vi "initializeKickForceValues.vi"(6 "samples":dbl, 7 "kickforce_min":dbl=1.0, 8 "error in (no error)":errorcluster, 9 "kickforce_max":dbl, 10 "delta":dbl, 11 "Game in":refnum<class "Game.lvclass">) -> (0 "error out":errorcluster, 2 "kickForceList":dbl[][](array[numeric]), 3 "Game out":refnum<class "Game.lvclass">)   [LabVIEW 2021, in "Game.lvclass"]
uses:
  Game.lvclass
  <vilib>/Analysis/1siggen.llb/Ramp Pattern by Delta.vi
  <vilib>/Analysis/NI_AALBase.lvlib
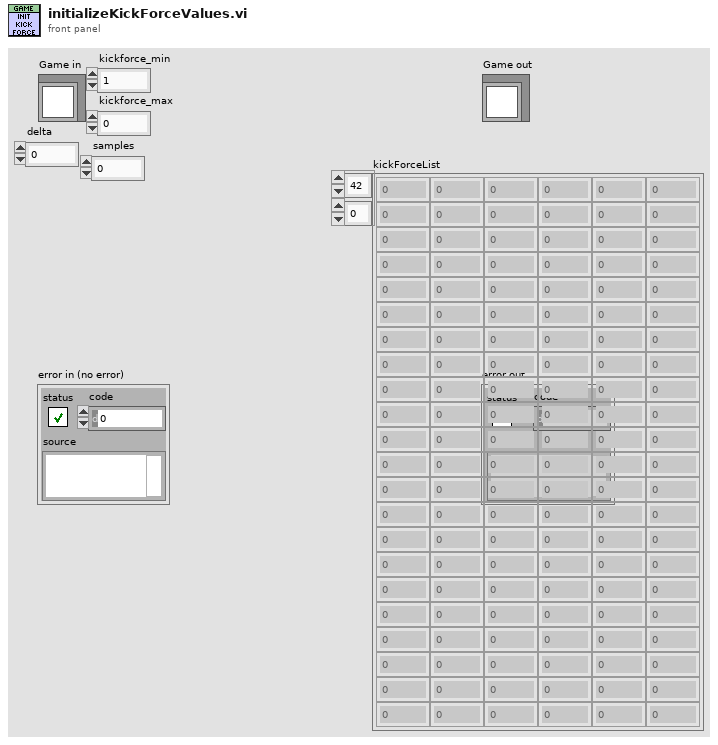
[diagram p1: front panel]
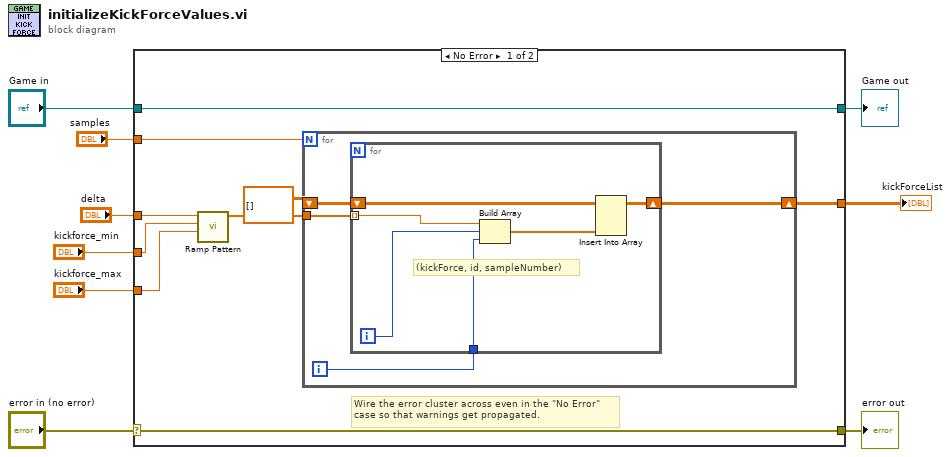
[diagram p0: block diagram]
diagram:
  n1 = case shown="No Error" "error in (no error)" {
    selector: "error in (no error)" -> [w17 w30]
    tunnel: [w17 w30] -> w8
    tunnel: [w18 w29] -> w6
    tunnel: "Game in" -> [w18 w29]
    tunnel: "delta" -> [w16 _]
    tunnel: "kickforce_min" -> [w15 _]
    tunnel: "kickforce_max" -> [w14 _]
    tunnel: "samples" -> [w12 _]
    tunnel: [w10 _] -> w1
    frame No Error {
      # "Wire the error cluster across even in the \"No Error\"\ncase so that warnings get propagated."
      n2 = call-poly <vilib>:"Ramp Pattern.vi"("start"=w14, "end"=w15, "delta"=w16) -> ("Ramp Pattern"=w13:dbl[])  [unwired: 6 in, 2 out]
      n3 = for {
        N: w12 -> [_]
        tunnel: w13 -> [w22]
        shift-right: [w20] -> w10
        shift-left: dbl[][] [] -> [w19]
        i -> [w21]
        n4 = for {
          tunnel: w22 -> [w28] mode=indexing
          tunnel: w21 -> [w26]
          shift-right: [w24] -> w20
          shift-left: w19 -> [w23]
          i -> [w27]
          # "(kickForce, id, sampleNumber)"
          n5 = Build Array(w28, w27, w26) -> (w25:dbl[])
          n6 = Insert Into Array(array=w23, new element=w25) -> (w24:dbl[][])  [unwired: 2 in]
        }
      }
    }
    frame Error {
    }
  }
  "error out" <- w8
  "Game out" <- w6
  "kickForceList" <- w1
